vi "Initialise-IO.vi"(8 "error in (no error)":errorcluster, 10 "Multicolumn Listbox":refnum<vi>, 11 "MulColLBTable.lvclass":refnum<class "MulColLBTable.lvclass">) -> (0 "error out":errorcluster, 3 "MulColLBTable.lvclass out":refnum<class "MulColLBTable.lvclass">)   [LabVIEW 2020, in "MulColLBTable.lvclass"]
uses:
  MulColLBTable.lvclass
  MulColLBTable.lvclass/MulColLBTable.ctl
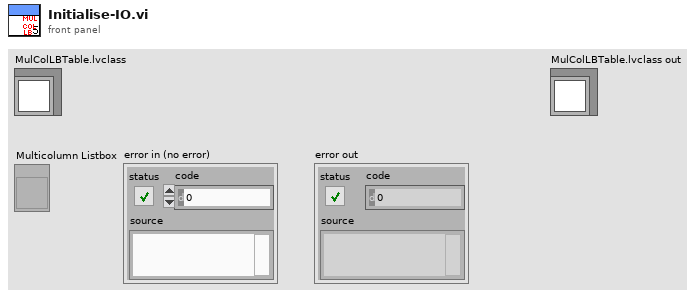
[diagram p1: front panel]
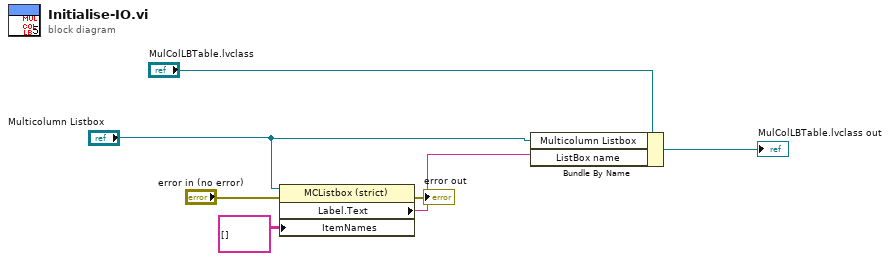
[diagram p0: block diagram]
diagram:
  n1 = property class="MCListbox (strict)"(reference="Multicolumn Listbox", error in="error in (no error)", "ItemNames"=string[][] [] ("Item Names")) -> (error out=→"error out":errorcluster, "Label.Text"=w6:string)  [unwired: 1 out]
  n2 = Bundle By Name(cluster="MulColLBTable.lvclass", "Multicolumn Listbox"="Multicolumn Listbox", "ListBox name"=w6) -> (→"MulColLBTable.lvclass out":refnum<class "MulColLBTable.lvclass">)
